vi "Configure Trigger Slope [TS].vi"(8 "error in (no error)":errorcluster, 10 "trigger slope (0: Positive)":i32(ring) items=["Positive", "Negative"], 11 "CS++DMM in":refnum<class "CS++DMM.lvclass">) -> (0 "error out":errorcluster, 3 "CS++DMM out":refnum<class "CS++DMM.lvclass">)   [LabVIEW 2016, in "CS++DMM.lvlib" / "CS++DMM.lvclass"]
doc: "This VI configures the polarity of the external trigger source of the DMM.\n\nNote:\n\n(1) This VI is part of the IviDmmTriggerSlope [TS] extension group."
uses:
  CS++DMM.lvclass
  CSPP_Core/Classes/CS++ProcessVariables/ProcessVariable/PV.lvclass
  PV-Enum.ctl
  CSPP_Core/Classes/CS++ProcessVariables/ProcessVariable/PV.lvclass/PV.ctl
  CS++DMM.lvclass/CS++DMM.ctl
  CSPP_Core/Classes/CS++ProcessVariables/ProcessVariable/Write Data.vi
  CSPP_Core/Classes/CS++ProcessVariables/ProcessVariable/Write Timestamp.vi
  CSPP_Core/Classes/CS++ProcessVariables/ProcessVariable/Write Quality.vi
  CSPP_Core/Classes/CS++ProcessVariables/ProcessVariable/Write status.vi
  CSPP_Core/Classes/CS++ProcessVariables/PVConnection/PVConnection.lvclass
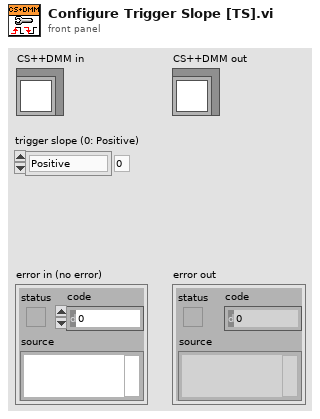
[diagram p1: front panel]
types:
  T1 = typedef "CS++DMM.lvlib/CS++DMM.lvclass/PV-Enum.ctl" = enum16{"AbsoluteResolution", "ACMaxFrequency", "ACMinFrequency", "ActualRange", "Alpha", "ApertureTime", "FixedReferenceJunction", "FrequencyVoltageRange", "PowerLineFrequency", "Range", "Reading", "Resistance", "SampleInterval", "TriggerDelay", "ApertureTimeUnit", "AutoZeroMode", "MeasCompleteDestination", "MeasurementFunction", "ReferenceJunctionType", "SampleCount", "SampleTrigger", "ThermocoupleType", "TransducerType", "TriggerCount", "TriggerSlope", "TriggerSource", "MPReading", "IsOverRange"}
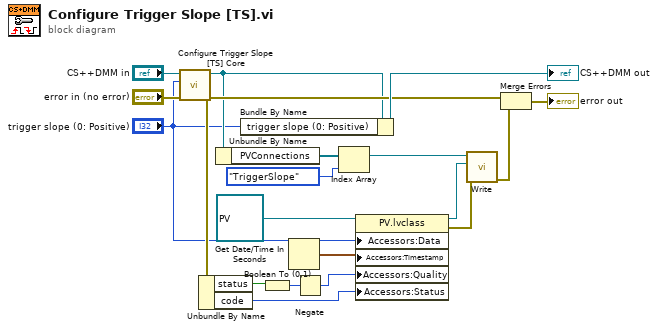
[diagram p0: block diagram]
diagram:
  n1 = call-dynamic "Configure Trigger Slope [TS] Core.vi"("error in (no error)"="error in (no error)", "trigger slope (0: Positive)"="trigger slope (0: Positive)", "CS++DMM in"="CS++DMM in") -> ("error out"=w7:errorcluster, "CS++DMM out"=w6:refnum<class "CS++DMM.lvclass">)  [unwired: 7 in]
  n2 = Unbundle By Name(w7) -> ("status"=w15:bool, "code"=w12:i32)
  n3 = Unbundle By Name(w6) -> ("PVConnections"=w10:refnum<class "PVConnection.lvclass">[])
  n4 = Bundle By Name(cluster=w6, "trigger slope (0: Positive)"="trigger slope (0: Positive)") -> (→"CS++DMM out":refnum<class "CS++DMM.lvclass">)
  n5 = Boolean To (0,1)(Boolean=w15) -> (0, 1=w14:i16)
  n6 = Get Date/Time In Seconds() -> (seconds since 1Jan1904=w11:timestamp)
  n7 = Negate(x=w14) -> (-x=w13:i16)
  n8 = Index Array(array=w10, index=PV-Enum."TriggerSlope" ("PV-Enum")) -> (element=w2:refnum<class "PVConnection.lvclass">)
  n9 = property class="PV.lvclass"(reference=refnum<class "PV.lvclass"> refnum ("CS++ProcessVariables.lvlib:PV.lvclass"), "Accessors:Data"="trigger slope (0: Positive)", "Accessors:Timestamp"=w11, "Accessors:Quality"=w13, "Accessors:Status"=w12) -> (reference out=w9:refnum<class "PV.lvclass">, error out=w8:errorcluster)  [unwired: 1 in]
  n10 = call "Write.vi"("error in (no error)"=w8, "PV"=w9, "PVConnection in"=w2) -> ("error out"=w3:errorcluster)  [unwired: 7 in, 1 out]
  n11 = Merge Errors(w7, w3) -> (→"error out":errorcluster)
